vi "LT_init.vi"(7 "do_reset":bool=TRUE, 8 "error in":errorcluster, 9 "Converter Type\n(180: Turbovac 350/450 i)":T3=187 items=["Turbovac 350/450 i"=180, "Turbovac 350/450 i with optional interface"=181, "Turbovac 350/450 iX"=182, "Turbovac 90/250 i"=190, "Turbovac 90/250 with optional interface"=191, "Turbovac 90/250 iX"=192, "TURBOVAC 850/950 i"=195, "TURBOVAC 850/950 i with optional interface"=196, "TURBOVAC 850/950 iX"=197, "TURBOVAC 1300 i"=185, "TURBOVAC 1300 i with optional interface"=186, "TURBOVAC 1300 iX"=187], 10 "Converter address (0)":u8, 11 "VISA in":refnum<visa-resource-name>="COM43") -> (0 "error out":errorcluster, 2 "dev_param_out":T1={"Length of data block"=14, "Converter address"=0, "Converter type"=180, "PZD1"=0, "PZD2"=0} {"Converter type" items=["Turbovac 350/450 i"=180, "Turbovac 350/450 i with optional interface"=181, "Turbovac 350/450 iX"=182, "Turbovac  90/250 i"=190, "Turbovac  90/250 with optional interface"=191, "Turbovac  90/250 iX"=192, "Turbovac  850/950 i"=195, "Turbovac  850/950 i with optional interface"=196, "Turbovac  850/950 iX"=197, "Turbovac 1350/1450 i"=185, "Turbovac 1350/1450 i with optional interface"=186, "Turbovac 1350/1450 iX"=187]; "Length of data block" items=["14"=14, "22"=22]}, 3 "VISA out":refnum<visa-resource-name>)   [LabVIEW 2019]
doc: "Example VI to demonstrate the use of the Oerlikon Leybold TMP driver."
uses:
  <instrlib>/Leybold TURBOVAC/Public/Ctl/Converter Type Control.ctl
  <instrlib>/Leybold TURBOVAC/Public/Ctl/Device Parameters Indicator.ctl
  <instrlib>/Leybold TURBOVAC/Public/Ctl/Converter Type Indicator.ctl
  <instrlib>/Leybold TURBOVAC/Leybold TURBOVAC.lvlib
panel:
  # "The converter address and type don't matter\nsince we use the remote drive unit (iR) via USB."
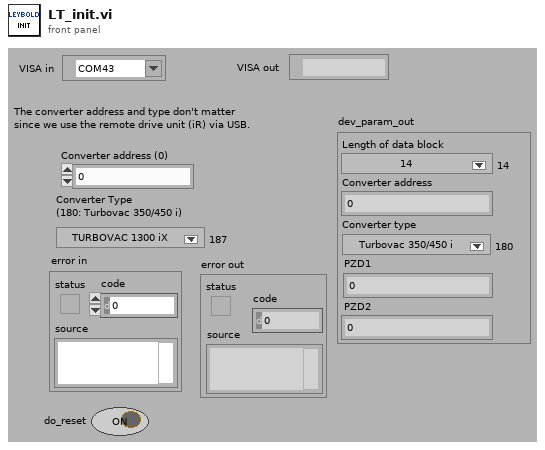
[diagram p1: front panel]
types:
  T1 = typedef "Leybold TURBOVAC.lvlib/Device Parameters Indicator.ctl" = cluster{"Length of data block":u8, "Converter address":u8, "Converter type":T2, "PZD1":u16, "PZD2":u16}
  T2 = typedef "Leybold TURBOVAC.lvlib/Converter Type Indicator.ctl" = u16
  T3 = typedef "Leybold TURBOVAC.lvlib/Converter Type Control.ctl" = u16
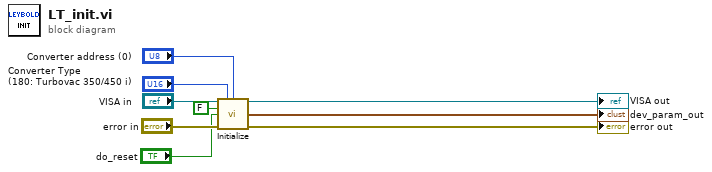
[diagram p0: block diagram]
diagram:
  n1 = call <instrlib>:"Initialize.vi"("VISA resource name"="VISA in", "Converter Type\n(180: Turbovac 350/450 i)"="Converter Type\n(180: Turbovac 350/450 i)", "Converter address (0)"="Converter address (0)", "ID Query? (T: Yes)"=FALSE, "Reset? (T: Yes)"="do_reset", "error in (no error)"="error in") -> ("VISA resource name out"=→"VISA out":refnum<visa-resource-name>, "Device parameters out"=→"dev_param_out":T1, "error out"=→"error out":errorcluster)  [unwired: 7 in]
